vi "rx_adc.vi"(9 "VISA resource name":refnum<visa-resource-name>="COM3", 11 "error in":errorcluster) -> ()   [LabVIEW 2015]
uses:
  <vilib>/Instr/_visa.llb/VISA Configure Serial Port (Instr).vi
  <instrlib>/Rohde&Schwarz RF Signal Generator/Rohde&Schwarz RF Signal Generator.lvlib
panel:
  out "parameters_b":dbl[](array[numeric])
  in  "VISA resource name 2":refnum<visa-resource-name>="GPIB0::28::INSTR" caption="VISA resource name"
  in  "R&S SMA100":refnum<visa-resource-name>="GPIB0::10::INSTR"
  in  "cnt/setp":enum16{"SETP", "COUNT"}(ring)=enum."COUNT"
  out "Freq_Tab":u32[](array[numeric])
  in  "EABLE Insert":bool
  in  "Insert Point":u32
  in  "Value":u32=3 caption="Point Num"
  in  "freq_max(Mhz)":u32=2300
  in  "freq_min(Mhz)":u32=2200
  in  "OK Button":bool
  in  "stop":bool
  in  "Tab Control":enum32{"A通道频谱", "B通道频谱"}(tab)
  out "XY Graph":cluster{dbl[], dbl[]}(graph)
  out "XY Graph 2":cluster{dbl[], dbl[]}(graph)
  out "vol20":string
  out "vol13":string
  out "frequency":string
  out "spectrum_a":dbl[](array[numeric])
  out "fre_a":dbl[](array[numeric])
  out "parameters_a":dbl[](array[numeric])
  out "dBFS_a":dbl
  out "snr_a":dbl
  out "sfdr_a":dbl
  out "sinad_a":dbl
  out "thd_a":dbl
  out "enob_a":dbl
  out "offset_a":dbl
  in  "图片保存路径":path=path "C:/Users/pigandhome/Desktop/Everst_LV2015/Everst_TestReport/Screenshot/RX"
  in  "fifo文件路径":path=path "E:/fifo.txt"
  in  "SPUR340 2":dbl=1.0
  in  "DATA_IQ 2":dbl=1.0
  in  "DATA_LOAD 2":dbl=1.0
  in  "DATA_WRITE 2":dbl=1.0
  in  "NF_TEST 2":dbl
  in  "FFT 2":dbl=1.0
  in  "ANALYZE_INL 2":dbl
  in  "ANALYZE_SPECTRUM 2":dbl=1.0
  in  "NCO 2":dbl=1.0
  in  "CHB":dbl
  out "VISA resource name out":refnum<visa-resource-name>
  in  "FPGA_PHASE":dbl
  in  "LVDS_SELF":dbl
  in  "LOOP_TEST":dbl
  in  "ADC_ONLY":dbl
  in  "STG2":dbl
  in  "STG1":dbl
  in  "CAP_MISMATCH":dbl
  in  "COMP_TRIM":dbl=1.0
  in  "MANUAL_TRIM":dbl=1.0
  in  "PROBE":dbl
  in  "CONFIG_DC":dbl=1.0
  in  "HIZ_INPUT":dbl=1.0
  in  "NCO":dbl=1.0
  in  "CONFIG":bool
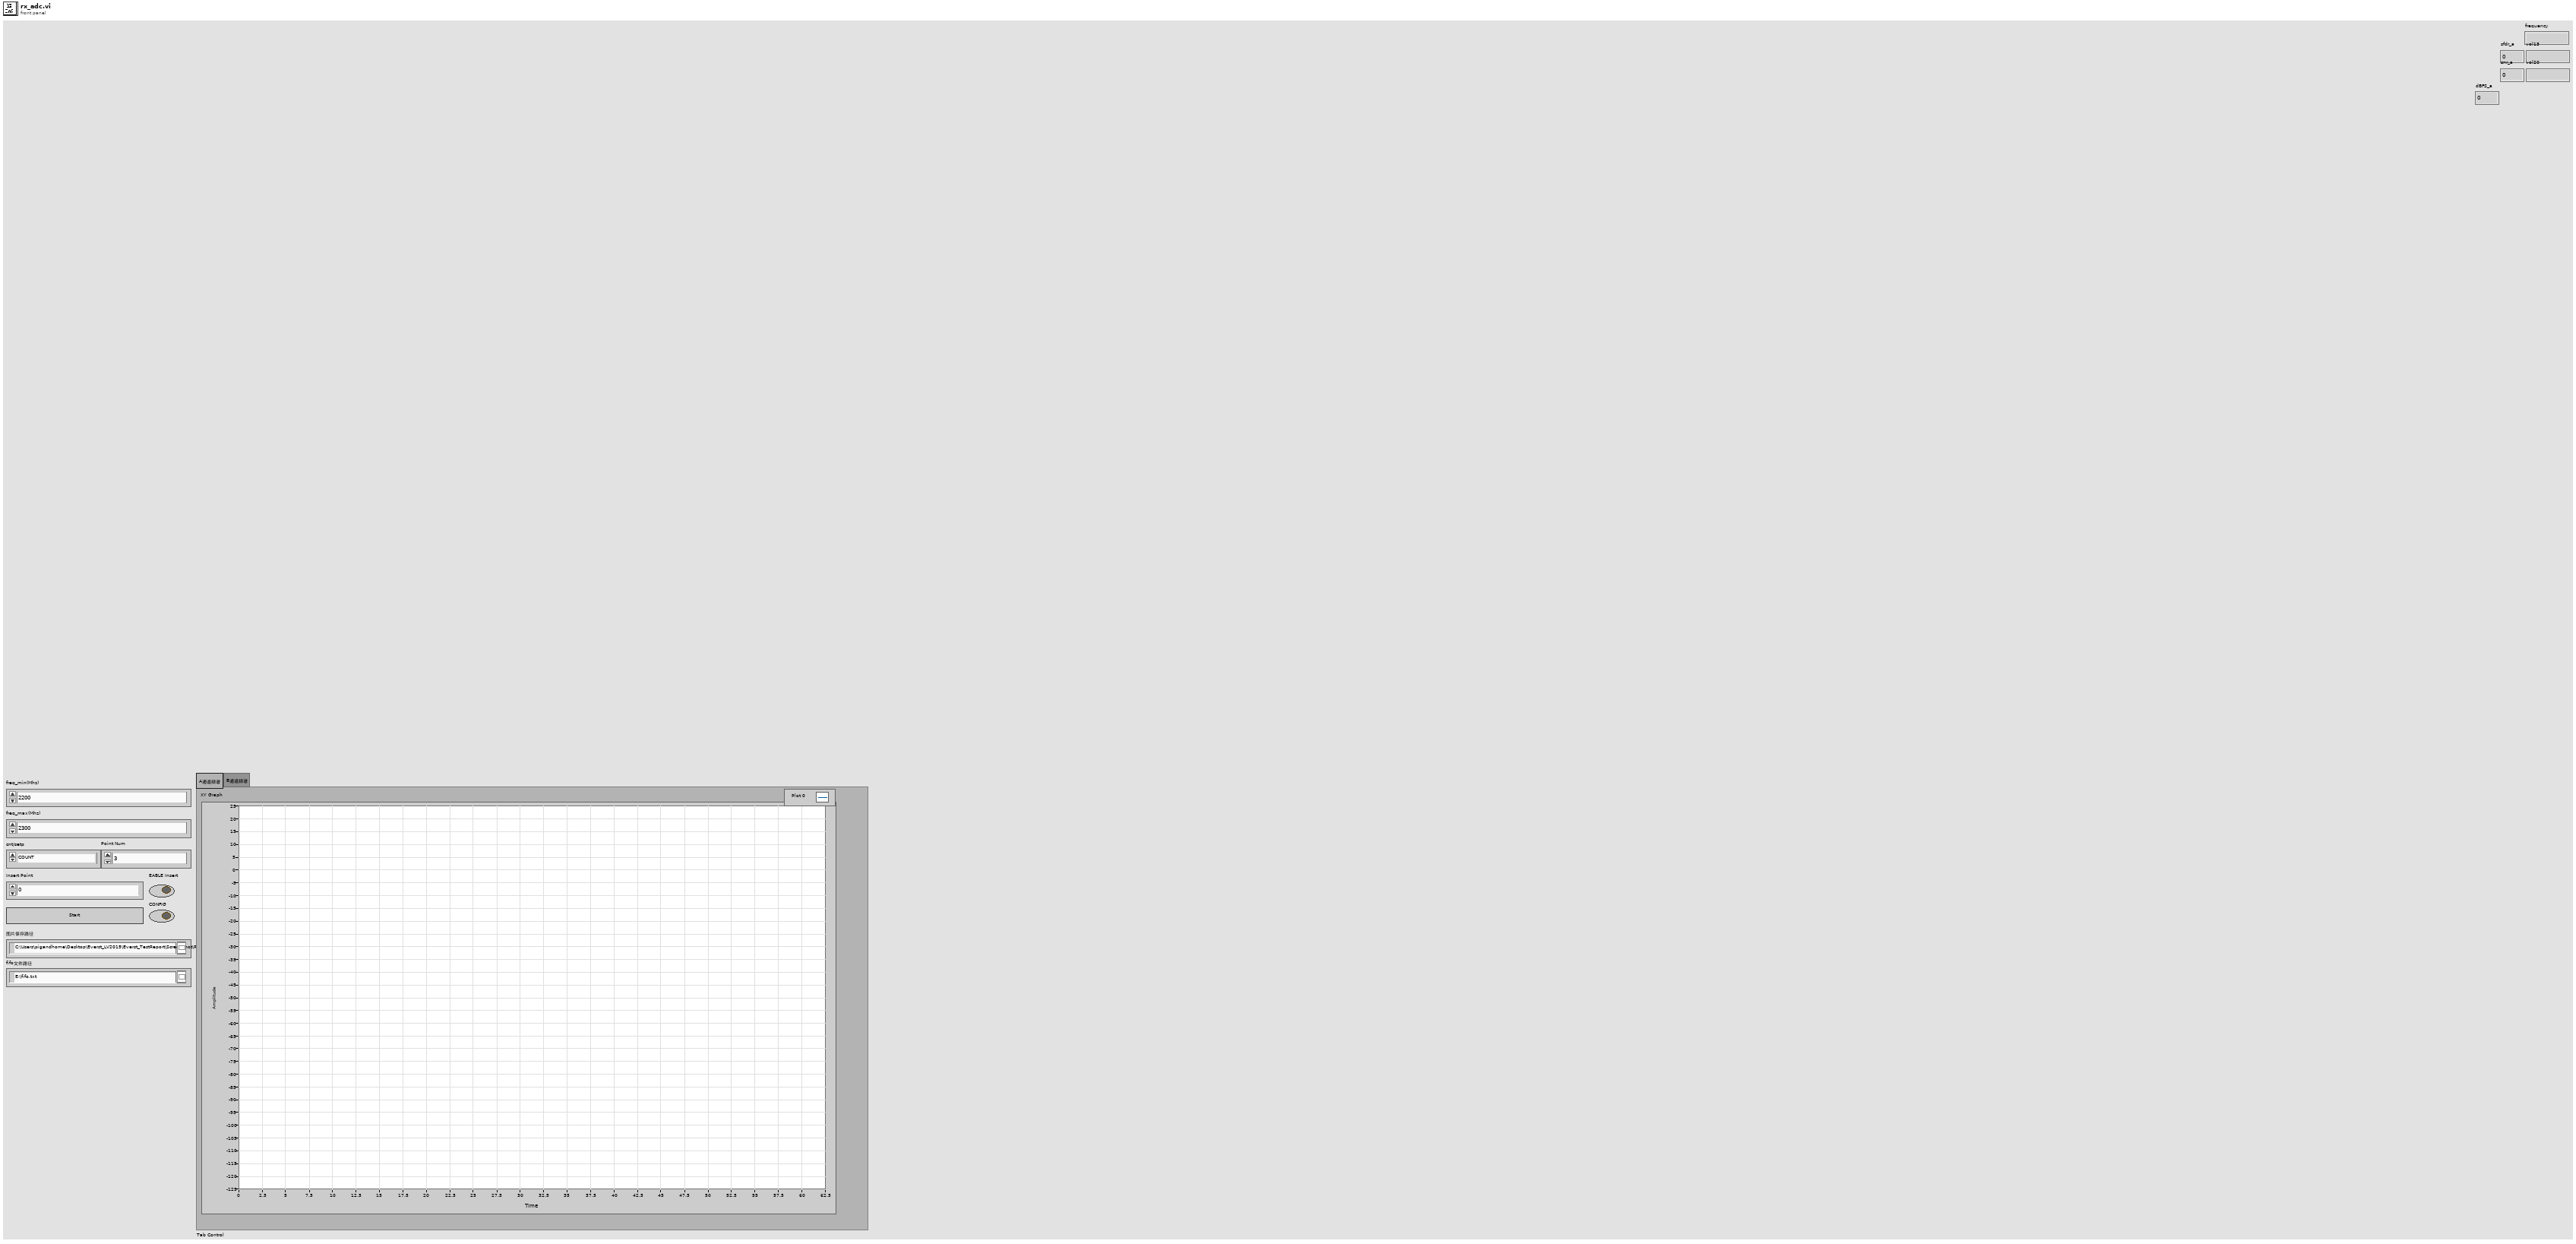
[diagram p1: front panel]
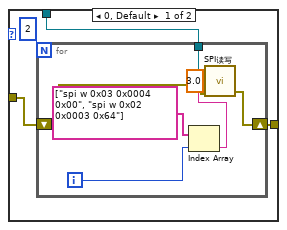
[diagram p3: hidden frame]
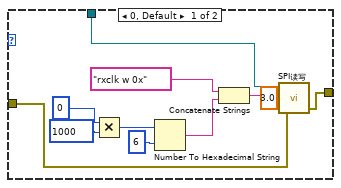
[diagram p4: hidden frame]
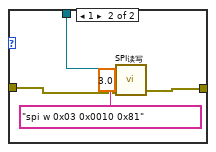
[diagram p5: hidden frame]
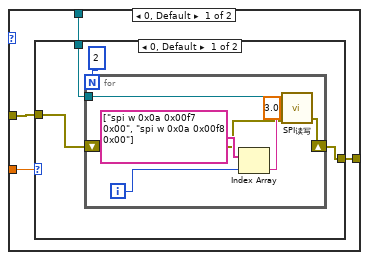
[diagram p6: hidden frame]
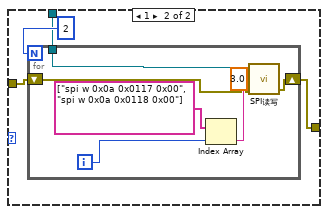
[diagram p7: hidden frame]
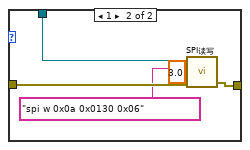
[diagram p10: hidden frame]
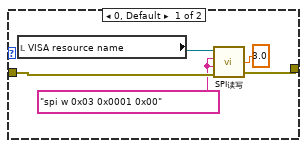
[diagram p12: hidden frame]
diagram:
  w39 = u16 0 items=["无", "XON/XOFF", "RTS/CTS", "XON/XOFF & RTS/CTS", "DTR/DSR", "XON/XOFF & DTR/DSR"] ("flow control (0:none)")
  w40 = u16 10 items=["1.0"=10, "1.5"=15, "2.0"=20] ("stop bits (10: 1 bit)")
  n1 = call-poly "VISA Configure Serial Port"("VISA resource name"="VISA resource name", "baud rate (9600)"=u32 921600, "data bits (8)"=u16 8, "parity (0:none)"=enum16{"None", "Odd", "Even", "Mark", "Space"}."None", "error in (no error)"="error in", "stop bits (10: 1 bit)"=w40, "flow control (0:none)"=w39) -> ("VISA resource name out"=w38:refnum<visa-resource-name>, "error out"=w37:errorcluster)  [unwired: 7 in]
  "VISA resource name out" <- w38
  n2 = VISA Clear(VISA resource name=w38, error in (no error)=w37) -> (VISA resource name out=w34:refnum<visa-resource-name>, error out=w15:errorcluster)
  n3 = call <instrlib>:"RSSMA Initialize.vi"("error in (no error)"=w15, "Resource Name (GPIB::28)"="R&S SMA100") -> ("error out"=w21:errorcluster, "dup VISA session"=w23:refnum<visa-resource-name>)  [unwired: 8 in]
  n4 = call <instrlib>:"RSSMA Configure RF Frequency.vi"("error in (no error)"=w21, "VISA session"=w23) -> ("error out"=w20:errorcluster, "dup VISA session"=w24:refnum<visa-resource-name>)  [unwired: 8 in]
  n5 = call <instrlib>:"RSSMA Configure Fixed RF Level.vi"("VISA session"=w24, "Amplitude (-30.0 dBm)"=-50.0, "error in (no error)"=w20) -> ("dup VISA session"=w18:refnum<visa-resource-name>, "error out"=w19:errorcluster)  [unwired: 11 in]
  n6 = call <instrlib>:"RSSMA Set Output State.vi"("error in (no error)"=w19, "RF Output State (F: Off)"=TRUE, "VISA session"=w18) -> ("error out"=w13:errorcluster, "dup VISA session"=w5:refnum<visa-resource-name>)  [unwired: 7 in]
  n7 = call <instrlib>:"Initialize.vi"("VISA resource name"="VISA resource name 2", "error in (no error)"=w13) -> ("VISA resource name out"=w11:refnum<visa-resource-name>, "error out"=w12:errorcluster)  [unwired: 12 in]
  n8 = call <instrlib>:"Configure RF.vi"("Power Level (-30.0)"=-50.0, "error in"=w12, "Frequency (1.0e9)"=2000000000.0, "VISA resource name"=w11) -> ("error out"=w10:errorcluster, "VISA resource name out"=w9:refnum<visa-resource-name>)  [unwired: 6 in]
  n9 = call <instrlib>:"Configure Output Enabled.vi"("error in"=w10, "Output Enabled (Off)"=TRUE, "VISA resource name"=w9) -> ("error out"=w6:errorcluster, "VISA resource name out"=w4:refnum<visa-resource-name>)  [unwired: 7 in]
  n10 = call "Set_Freq_Table.vi"("EABLE Insert"="EABLE Insert", "Insert Point"="Insert Point", "Value"="Value", "cnt/setp"="cnt/setp", "freq_max(Mhz)"="freq_max(Mhz)", "freq_min(Mhz)"="freq_min(Mhz)") -> ("Freq_Tab"=w2:u32[])
  "Freq_Tab" <- w2
  n11 = Array Size(array=w2) -> (size(s)=w25:i32)
  n12 = while {
    tunnel: w34 -> [w53]
    tunnel: w6 -> [w52]
    tunnel: "fifo文件路径" -> [w50]
    tunnel: "图片保存路径" -> [w49]
    tunnel: w25 -> [w48]
    tunnel: w5 -> [w47]
    tunnel: w4 -> [w46]
    tunnel: w2 -> [w45]
    tunnel: path "C:/Users/pigandhome/Desktop/Everst_LV2015/Everst_TestReport/EVERST_TestReport_#  4_20171014120206.xlsx" ("path") -> [w44]
    stop <- "stop" stop-if-true
    n13 = event shown="[0] \"OK Button\": Value Change" {
      selector: _ -> [_]
      dyn-events: _ -> [_]
      timeout: _ -> [_]
      tunnel: w53 -> [w75]
      tunnel: w52 -> [w74]
      tunnel: w50 -> [w71]
      tunnel: w49 -> [w70]
      tunnel: w48 -> [w69]
      tunnel: w47 -> [w67]
      tunnel: w46 -> [w66]
      tunnel: w45 -> [w60]
      tunnel: w44 -> [w55]
      event "OK Button": Value Change {
        n14 = event-data() -> ()  [unwired: 1 in, 6 out]
        n15 = local read "NCO"() -> (w80:dbl)
        n16 = case shown="1" w80 {
          tunnel: w74 -> [w279 w284]
          tunnel: [w278 w282] -> w76
          frame 0, Default {
            w277 = "spi w 0x03 0x0001 0x00" ("往芯片写数据")
            n17 = local read "VISA resource name"() -> (w280:refnum<visa-resource-name>)
            n18 = call "SPI读写.vi"("DELAY"=3.0, "error in (no error)"=w279, "从芯片读数据"=w277, "往芯片写数据"=w277, "VISA resource name"=w280) -> ("error out"=w278:errorcluster)  [unwired: 1 out]
          }
          frame 1 {
            n19 = local read "VISA resource name"() -> (w285:refnum<visa-resource-name>)
            n20 = call "SPI读写.vi"("DELAY"=3.0, "error in (no error)"=w284, "往芯片写数据"="spi w 0x03 0x0001 0x80", "VISA resource name"=w285) -> ("error out"=w282:errorcluster)  [unwired: 1 in, 1 out]
          }
        }
        n21 = local read "CONFIG"() -> (w77:bool)
        n22 = case shown="True" w77 {
          tunnel: w76 -> [w143 _]
          tunnel: [w143 w166] -> w78
          tunnel: [w142 w144] -> w79
          tunnel: w75 -> [w142 w144]
          frame False {
          }
          frame True {
            w146 = string[] ["spi w 0x08 0x0001 0xe0", "spi w 0x03 0x0005 0x00", "spi w 0x04 0x0000 0x00", "spi w 0x04 0x0001 0x00", "spi w 0x04 0x0002 0x00", "spi w 0x04 0x0000 0x44", "spi w 0x04 0x0001 0x60", "spi w 0x04 0x0002 0x00", "spi w 0x04 0x0005 0x76", "spi w 0x04 0x0006 0x67", "spi w 0x04 0x0007 0x66", "spi w 0x05 0x000e 0x40", "spi w 0x04 0x001c 0x20", "spi w 0x05 0x0003 0xe0", "spi w 0x05 0x0004 0x1f", "spi w 0x05 0x000a 0x20", "spi w 0x05 0x0008 0xe2", "spi w 0x05 0x0008 0xea", "spi w 0x05 0x0015 0x20", "spi w 0x05 0x0016 0x12", "spi w 0x05 0x001c 0x20", "spi w 0x05 0x001a 0xc2", "spi w 0x05 0x001a 0xca", "spi w 0x06 0x000a 0x00", "spi w 0x06 0x0010 0x00", "spi w 0x0a 0x0132 0x5b", "spi w 0x08 0x0012 0x5b", "spi w 0x0a 0x0133 0x71", "spi w 0x08 0x0013 0x71", "spi w 0x06 0x000b 0x3a", "spi w 0x06 0x0003 0x03", "spi w 0x06 0x0009 0xC6", "spi w 0x06 0x0006 0x53", "spi w 0x06 0x0007 0x2E"] ("output array")
            n23 = Array Size(array=w146) -> (size(s)=w148:i32)
            n24 = for {
              N: w148 -> [_]
              tunnel: w146 -> [w173]
              tunnel: w144 -> [w168]
              shift-right: [w167] -> w145
              shift-left: _ -> [w170]
              i -> [w172]
              n25 = Index Array(array=w173, index=w172) -> (element=w171:string)
              n26 = call "SPI读写.vi"("DELAY"=3.0, "error in (no error)"=w170, "从芯片读数据"=w171, "往芯片写数据"=w171, "VISA resource name"=w168) -> ("error out"=w167:errorcluster)  [unwired: 1 out]
            }
            n27 = local read "CONFIG_DC"() -> (w165:dbl)
            n28 = case shown="1" w165 {
              tunnel: w145 -> [w272 w275]
              tunnel: w144 -> [_ w274]
              tunnel: [w272 w273] -> w163
              frame 0, Default {
              }
              frame 1 {
                n29 = call "everest_adc_bias_init.vi"("error in"=w275, "VISA resource name"=w274) -> ("error out"=w273:errorcluster)  [unwired: 9 in]
              }
            }
            n30 = local read "HIZ_INPUT"() -> (w164:dbl)
            n31 = case shown="0, Default" w164 {
              tunnel: w144 -> [w265 w271]
              tunnel: w163 -> [w266 w270]
              tunnel: [w263 w268] -> w161
              frame 0, Default {
                n32 = call "SPI读写.vi"("DELAY"=3.0, "error in (no error)"=w266, "往芯片写数据"="spi w 0x0a 0x0130 0x04", "VISA resource name"=w265) -> ("error out"=w263:errorcluster)  [unwired: 1 in, 1 out]
              }
              frame 1 {
                n33 = call "SPI读写.vi"("DELAY"=3.0, "error in (no error)"=w270, "往芯片写数据"="spi w 0x0a 0x0130 0x06", "VISA resource name"=w271) -> ("error out"=w268:errorcluster)  [unwired: 1 in, 1 out]
              }
            }
            n34 = local read "MANUAL_TRIM"() -> (w162:dbl)
            n35 = case shown="1" w162 {
              tunnel: "CHB" -> [_ w260]
              tunnel: w161 -> [w257 w261]
              tunnel: w144 -> [_ w259]
              tunnel: [w257 w258] -> w159
              frame 0, Default {
              }
              frame 1 {
                n36 = call "everest_adc_manul_trim.vi"("error in (no error)"=w261, "CHB"=w260, "VISA resource name"=w259) -> ("error out"=w258:errorcluster)
              }
            }
            n37 = local read "CAP_MISMATCH"() -> (w160:dbl)
            n38 = local read "STG2"() -> (w157:dbl)
            n39 = local read "STG1"() -> (w158:dbl)
            n40 = case shown="1" w160 {
              tunnel: w159 -> [w250 w256]
              tunnel: w144 -> [_ w255]
              tunnel: "CHB" -> [_ w254]
              tunnel: w158 -> [_ w253]
              tunnel: w157 -> [_ w252]
              tunnel: [w250 w251] -> w155
              frame 0, Default {
              }
              frame 1 {
                n41 = call "everest_adc_cap_mismatch.vi"("STG2"=w252, "STG1"=w253, "error in (no error)"=w256, "CHB"=w254, "VISA resource name"=w255) -> ("error out"=w251:errorcluster)
              }
            }
            n42 = local read "COMP_TRIM"() -> (w156:dbl)
            n43 = case shown="1" w156 {
              tunnel: [w220 w247] -> w153
              tunnel: "CHB" -> [w223 w249]
              tunnel: w144 -> [w222 w248]
              tunnel: w155 -> [w221 w246]
              frame 0, Default {
                n44 = case shown="0, Default" w223 {
                  tunnel: w222 -> [w227 w237]
                  tunnel: w221 -> [w226 w235]
                  tunnel: [w225 w236] -> w220
                  frame 0, Default {
                    n45 = for {
                      N: 2 -> [_]
                      tunnel: w227 -> [w231]
                      shift-right: [w229] -> w225
                      shift-left: w226 -> [w230]
                      i -> [w234]
                      n46 = Index Array(array=string[] ["spi w 0x0a 0x00f7 0x00", "spi w 0x0a 0x00f8 0x00"], index=w234) -> (element=w232:string)
                      n47 = call "SPI读写.vi"("DELAY"=3.0, "error in (no error)"=w230, "往芯片写数据"=w232, "VISA resource name"=w231) -> ("error out"=w229:errorcluster)  [unwired: 1 in, 1 out]
                    }
                  }
                  frame 1 {
                    n48 = for {
                      N: 2 -> [_]
                      shift-right: [w241] -> w236
                      shift-left: w235 -> [w242]
                      tunnel: w237 -> [w240]
                      i -> [w245]
                      n49 = Index Array(array=string[] ["spi w 0x0a 0x0117 0x00", "spi w 0x0a 0x0118 0x00"], index=w245) -> (element=w243:string)
                      n50 = call "SPI读写.vi"("DELAY"=3.0, "error in (no error)"=w242, "往芯片写数据"=w243, "VISA resource name"=w240) -> ("error out"=w241:errorcluster)  [unwired: 1 in, 1 out]
                    }
                  }
                }
              }
              frame 1 {
                n51 = call "everest_adc_comp_trim_init.vi"("CHB"=w249, "error in (no error)"=w246, "VISA resource name"=w248) -> ("error out"=w247:errorcluster)
              }
            }
            n52 = local read "LVDS_SELF"() -> (w154:dbl)
            n53 = case shown="0, Default" w154 {
              tunnel: w153 -> [w212 w218]
              tunnel: w144 -> [w213 w217]
              tunnel: [w211 w216] -> w151
              frame 0, Default {
                n54 = call "SPI读写.vi"("DELAY"=3.0, "error in (no error)"=w212, "往芯片写数据"="spi w 0x03 0x0010 0x80", "VISA resource name"=w213) -> ("error out"=w211:errorcluster)  [unwired: 1 in, 1 out]
              }
              frame 1 {
                n55 = call "SPI读写.vi"("DELAY"=3.0, "error in (no error)"=w218, "往芯片写数据"="spi w 0x03 0x0010 0x81", "VISA resource name"=w217) -> ("error out"=w216:errorcluster)  [unwired: 1 in, 1 out]
              }
            }
            n56 = local read "FPGA_PHASE"() -> (w152:dbl)
            n57 = case shown="1" w152 {
              tunnel: w151 -> [w191 w202]
              tunnel: w144 -> [w190 w201]
              tunnel: [w189 w200] -> w149
              frame 0, Default {
                n58 = Multiply(x=0, y=1000) -> (x*y=w196:i32)
                n59 = Number To Hexadecimal String(1:i16 6 ("宽度(-)"), 2:w196) -> (0:w193:string)
                n60 = Concatenate Strings("rxclk w 0x", w193) -> (w192:string)
                n61 = call "SPI读写.vi"("DELAY"=3.0, "error in (no error)"=w191, "往芯片写数据"=w192, "VISA resource name"=w190) -> ("error out"=w189:errorcluster)  [unwired: 1 in, 1 out]
              }
              frame 1 {
                n62 = Multiply(x=90, y=1000) -> (x*y=w207:i32)
                n63 = Number To Hexadecimal String(1:i16 6 ("宽度(-)"), 2:w207) -> (0:w204:string)
                n64 = Concatenate Strings("rxclk w 0x", w204) -> (w203:string)
                n65 = call "SPI读写.vi"("DELAY"=3.0, "error in (no error)"=w202, "往芯片写数据"=w203, "VISA resource name"=w201) -> ("error out"=w200:errorcluster)  [unwired: 1 in, 1 out]
              }
            }
            n66 = local read "LOOP_TEST"() -> (w150:dbl)
            n67 = case shown="1" w150 {
              tunnel: w149 -> [w176 w186]
              tunnel: w144 -> [w175 w187]
              tunnel: [w174 w185] -> w166
              frame 0, Default {
                n68 = for {
                  N: 2 -> [_]
                  tunnel: w175 -> [w180]
                  shift-right: [w179] -> w174
                  shift-left: w176 -> [w181]
                  i -> [w184]
                  n69 = Index Array(array=string[] ["spi w 0x03 0x0004 0x00", "spi w 0x02 0x0003 0x64"], index=w184) -> (element=w182:string)
                  n70 = call "SPI读写.vi"("DELAY"=3.0, "error in (no error)"=w181, "往芯片写数据"=w182, "VISA resource name"=w180) -> ("error out"=w179:errorcluster)  [unwired: 1 in, 1 out]
                }
              }
              frame 1 {
                n71 = call "everest_loop_test.vi"("error in (no error)"=w186, "VISA resource name"=w187) -> ("error out"=w185:errorcluster)
              }
            }
          }
        }
        n72 = VISA Close(VISA resource name=w79, error in (no error)=w78) -> (error out=w68:errorcluster)
        n73 = Path To String(path=w71) -> (string=w72:string)
        n74 = Path To String(path=w70) -> (string=w73:string)
        n75 = for {
          N: w69 -> [_]
          tunnel: w73 -> [w112]
          tunnel: w72 -> [w111]
          shift-right: [w110] -> _
          shift-left: w68 -> [w109]
          tunnel: w67 -> [w107]
          tunnel: w66 -> [w106]
          tunnel: [w87] -> w58 mode=indexing
          tunnel: [w83] -> w57 mode=indexing
          i -> [w104]
          n76 = local read "Freq_Tab"() -> (w105:u32[])
          n77 = local read "frequency"() -> (w126:string)
          n78 = local read "vol13"() -> (w127:string)
          n79 = local read "vol20"() -> (w128:string)
          n80 = Index Array(array=w105, index=w104) -> (element=w92:u32)
          n81 = Less?(x=w92, y=u32 2270) -> (x < y?=w88:bool)
          n82 = Boolean To (0,1)(Boolean=w88) -> (0, 1=w89:i16)
          n83 = Multiply(x=u32 1000000, y=w92) -> (x*y=w101:u32)
          n84 = call <instrlib>:"RSSMA Configure RF Frequency.vi"("error in (no error)"=w109, "Frequency (1.0e9 Hz)"=w101, "VISA session"=w107) -> ("error out"=w108:errorcluster)  [unwired: 7 in, 1 out]
          n85 = script code="if ANALYZE_SPECTRUM\n    fifo_len = 31;   %%% unit is k, 16/32/63\nelse\n    fifo_len = 16;   %%% unit is k\nend % ANALYZE_SPECTRUM\n%--------------------------------------------------------------------------\nfile = path;\n%--------------------------------------------------------------------------\n\nif CHB\n    file_captrim = 'chip2_chb_cap.mat';\nelse\n    file_captrim = 'chip2_cha_cap.mat';\nend % CHB\n%--------------------------------------------------------------------------\n\n%Initial s port\ns         = serial('COM3');     % need to change if com number changes\ns.InputBufferSize = 128e3;\nset(s,'BaudRate',921600);\nfopen(s);\n\n\nif ANALYZE_SPECTRUM\n\n    if DATA_WRITE\n%        fifo_data = fifo_read(s, fifo_len);\ncommand = sprintf('fifo rst\\n');\nfwrite(s, command);\nfprintf('%s',command);\npause(0.1);\ncommand = sprintf('fifo rst\\n');\nfwrite(s, command);\nfprintf('%s',command);\npause(0.1);\ncommand = sprintf('fifo status\\n');\nfwrite(s,command);\nfprintf('%s',command);\npause(0.03);\ncommand = sprintf('fifo wr\\n');\nfwrite(s,command);\npause(1);\ncommand = sprintf('fifo status\\n');\nfwrite(s,command);\npause(0.03);\ncommand = sprintf('fifo read 0x%s\\n',dec2hex(fifo_len,2));\nfwrite(s,command);\npause(0.03);\n\npause(0.03);\nnum1 = s.BytesAvailable;\n\ndata_buffer = int8(zeros(1,fifo_len*1e3*30+500));\nfprintf(1,'Read fifo(%dK).',fifo_len);\n\nii = 1;\nwhile num1 ~= 0\n    pause(0.1);    \n    read_data = fread(s, num1);\n    data_buffer(ii:ii+num1-1) = read_data';\n    ii = ii + num1;\n    num1 = s.BytesAvailable;\n    fprintf(1,'.');\n%     fprintf(1,'%d\\n',ii);\nend\n\nfprintf(1,'\\n');\nfifo_data = data_buffer;\n\n       fprintf(1,'---------------------Read fifo ok!------------------------------\\n');\n       fid = fopen(file,'w');\n       fprintf(fid,'%1c',fifo_data);\n       fclose(fid);\n    end\n\n    fclose(s);\n%--------------------------------------------------------------------------\n    if DATA_LOAD\n    % read from data file\n    fid      = fopen(file,'r');\n    temp     = fscanf(fid, '%s'); \n    len_temp = length(temp);\n\n    for ii = 1:1:3000\n       if strcmp(temp(ii:ii+9),'fiforead0x')\n           break;\n       end\n    end\n\n    temp1              = temp(ii+12:fifo_len*16*1024+ii+11);\n    num_of_samples     = length(temp1)/16;\n\n    samples_rising_a   = zeros(1,num_of_samples);\n    samples_falling_a  = zeros(1,num_of_samples);\n\n    samples_rising_b   = zeros(1,num_of_samples);\n    samples_falling_b  = zeros(1,num_of_samples);\n\n    for ii = 1:1:num_of_samples\n        temp_rising_a  = temp1(((ii-1)*16+1):((ii-1)*16+4));\n        temp_falling_a = temp1((ii-1)*16+5:(ii-1)*16+8);\n        temp_rising_b  = temp1((ii-1)*16+9:(ii-1)*16+12);\n        temp_falling_b = temp1((ii-1)*16+13:(ii-1)*16+16);\n\n        samples_rising_a(ii)   = hex2dec(temp_rising_a);\n        samples_falling_a(ii)  = hex2dec(temp_falling_a);\n        samples_rising_b(ii)   = hex2dec(temp_rising_b);\n        samples_falling_b(ii)  = hex2dec(temp_falling_b);\n\n        if samples_rising_a(ii) > 2^13-1\n            samples_rising_a(ii) = samples_rising_a(ii) - 2^14;\n        end\n\n        if samples_rising_b(ii) > 2^13-1\n            samples_rising_b(ii) = samples_rising_b(ii) - 2^14;\n        end\n\n        if samples_falling_a(ii) > 2^13-1\n            samples_falling_a(ii) = samples_falling_a(ii) - 2^14;\n        end\n\n        if samples_falling_b(ii) > 2^13-1\n            samples_falling_b(ii) = samples_falling_b(ii) - 2^14;\n        end\n    end\n\n    mean_rising_a   = round(mean(samples_rising_a));\n    mean_falling_a  = round(mean(samples_falling_a));\n    mean_rising_b   = round(mean(samples_rising_b));\n    mean_falling_b  = round(mean(samples_falling_b));\n    end \n\n    fclose all;\n%--------------------------------------------------------------------------\n\n% % plot data\n% figure('name','sampled waveform');\n% \n% subplot(2,2,1); \n% plot(samples_rising_a); \n% title('ADC VI output'); \n% grid on;\n% hold on;\n% \n% subplot(2,2,2);\n% plot(samples_falling_a);\n% title('ADC VQ output');\n% grid on;\n% hold on;\n% \n% subplot(2,2,3); \n% plot(samples_rising_b);\n% title('ADC HI output');\n% grid on;\n% hold on;\n% \n% subplot(2,2,4);\n% plot(samples_falling_b);\n% title('ADC HQ output');\n% grid on;\n% hold on;\n%--------------------------------------------------------------------------\n\n% do fft analysis\nif FFT\n\n    if CHB    % CHB\n        dataI = samples_rising_b';\n        dataQ = samples_falling_b';\n        \n        if NCO\n            if DATA_IQ\n                data  = dataI - j*dataQ;\n            else\n                data  = dataQ - j*dataI;\n            end\n        else\n            data  = dataQ;\n        end\n        \n    else      % CHA\n        dataI = samples_rising_a';\n        dataQ = samples_falling_a';\n   \n        if NCO\n            if DATA_IQ\n                data  = dataI - j*dataQ;\n            else\n                data  = dataQ - j*dataI;\n            end\n        else\n            data  = dataQ;\n        end\n    end\n\n    if NF_TEST\n        len  = length(data); \n        fs   = 125e6; \n        fsig = 5e6;\n        t    = 1/fs:1/fs:len/fs; \n        %sig  = 8191*cos(2*pi*t*fsig);\n        sig  = 8191*cos(2*pi*t*fsig) + j * 8191*cos(2*pi*t*fsig);\n        data = data + sig';\n    end\n    \n    if SPUR340\n        len  = length(data); \n        fs   = 125e6; \n        fsig = 20e6;\n        t    = 1/fs:1/fs:len/fs;\n        amp  = 8191 * 10^(-59.2198/20);\n        td   = 0 ;\n        phase = 0.0717;\n        %sig  = 8191*cos(2*pi*t*fsig);\n        sig  = amp*cos(2*pi*(t+td)*fsig+phase) - j * amp*sin(2*pi*(t+td)*fsig+phase);\n        win  = hanning(len);\n        data_fft  =  fft(data.*win);\n        sig_fft   =  fft(sig'.*win);\n        abs(data_fft(5244))\n        abs(sig_fft(5244))\n        angle(data_fft(5244))\n        angle(sig_fft(5244))\n        %data = data - sig';   \n    end\n    \n    save fftdata.dat data -ASCII\n\n%     Dynamics_14b_no_print;\n%Filename:   Dynamics_12b.m\n%Function:   Spectrum analaysis of 12b ADC\n%Author:     Maxgress\n%Date:       Dec. 2012\n%--------------------------------------------------------------------------\n\n%set constants\n%--------------------------------------------------------------------------\n\n%fsample  = 61.44e6*4;           % clock frequency\nfsample  = 500e6/4;           % clock frequency\nfsr      = 1;\n%numpts   = 131072*2;          % 128k data\nnumpts   = 4096;            % 128k data\nnumbits  = 14;              % 12bit \nsearch   = 1;                      \nnumharm  = 3;              % Number of harmonics \n\n\n%load data\n%--------------------------------------------------------------------------\n\n%load C:\\MG6802\\fftdata.dat;\n%load fftdata.dat\n\n%data     = fftdata;\n[a b]    = size(data);\nnumpts   = a;\nwindow   = 1;\ntwotone  = 0;\ndither   = 0;\n\n%dBFS     = 20*log10((max(real(data))-min(real(data)))/2^numbits);\ndBFS     = 10*log10(((max(real(data))-min(real(data)))/2^numbits)^2 + ((max(imag(data))-min(imag(data)))/2^numbits)^2);\n\ntmp1     = size(data);\ntmp1     = tmp1(1);\n\n%process data\n%--------------------------------------------------------------------------\n\nq        =  data;\nfbin     = (fsample/numpts);\t%this is the the FFT bin spacing\nVopp     =  max(q)-min(q);\t%this is the Peak-to-Peak ADC output\nVodbfs   =  20*log10(Vopp/2);\t%this is the ADC output in dBFS\nshift    =  (2^(numbits-1))-0.5;\nu        =  (q-shift)/shift;\n\nz        =   fft(u)/numpts;\n\n%%%%%%%%% Here are some magic windowing factors \n\nif window==1;\n   a0=0.3635819;\n   a1=0.4891775;\n   a2=0.1365995;\n   a3=0.0106411;\n   vec=0.5*[-a3 a2 -a1 2*a0 -a1 a2 -a3]*(numpts/2^numbits);\n   winh=conv(vec,z);\n   for i=1:numpts;\n\t\tz(i)=winh(i+3);\n   end;\n\t\t\nend;\nGwin=-20*log10(a0);\t     %this is the window's gain\n\n%%%%%%%%%  these simple transforms are how we use the fft result:\n\nvolts=abs(z(1:(numpts/2+1)));\n%volts(numpts/4:numpts/2+1)=0.00001;\n\npower=volts.^2;\ndbvolts=20*log10(2*volts+eps); % Why the factor of 2 applied to volts.\n%dbvolts(numpts/4:numpts/2+1)=-92;\nif window==1;\n\tdbvolts=dbvolts+Gwin;\t%this resets to normalized gain\nend;\ndbint=floor(dbvolts);\n\n%  if the oscillator frequencies are all over the place,\n%  we can go and find the input by looking for the max \n%  bin.  This is selected by the \"search\" flag.\n\nif search==1\n\ttempvolts=volts;\n\ttempvolts(1:4)=zeros(1,4);\n\t[a1,fund]=max(tempvolts);\n   finput=(fund-1)*fsample/numpts;\n   tempvolts(fund)=0;\n   if(twotone==1)\n      [a2,fundq]=max(tempvolts);\n      finputq=(fundq-1)*fsample/numpts;\n   end;   \nend;\n\n%%%%%%%%%%%%%  Now we analyze the results of the fft;\n%%%%%%%%%%%%%  If we know finput, we can find the harmonics:\nif(twotone==1)\nhq=0:(numharm-1);\nfhq=finputq*hq;\nrbinsq=round(fhq/(fsample/numpts));\nmultq=(floor(rbinsq/(numpts/2)));\npolq=(-1).^multq;\nactbinq=1+(numpts/2)*(1-polq)/2+polq.*(rbinsq-multq*numpts/2);\nfor i=1:numharm;\n      hdarrayq(i)=dbvolts(actbinq(i));\nend;\nend;\n\nh=0:(numharm-1);\nfh=finput*h;\nrbins=round(fh/(fsample/numpts));\nmult=(floor(rbins/(numpts/2)));\npol=(-1).^mult;\nactbin=1+(numpts/2)*(1-pol)/2+pol.*(rbins-mult*numpts/2);\ndbvoltsa=dbvolts;\n\nfor i=1:numharm;\n  \n      hdarray(i)=dbvolts(actbin(i));\n\nend;\n\n%%%%%%% After calculating harmonic bin locations, we can calculate the\n%%%%%%% noise floor for the SNR & SINAD. First exclude the power in the  \n%%%%%%% dither (this is the \"dither\" variable) band and the 50 individual\n%%%%%%% harmonic bins and the DC bin. An iterative approach is used.\n%%% actbin(1) is DC bin.  \n%%% actbin(2) is the fundamental.\n\nif dither>0\n\tpbins=power;\n\tstartBin=dither/fbin;\n\tavgpwr1=sum(pbins(startBin+1):pbins(startBin+5));\n\tfor i=1:startBin;\n\t\tpbins(i)=avgpwr1;\n\tend;\nelse\n\tpbins=power;\nend;\nsfdrarray=pbins;\nzeroset=0;\npowleng=1+length(power);\nvart=8;\nif window==0\n   \tfor i=1:numharm;\n         pbins(actbin(i))=0;\n         if(twotone==1)\n            pbins(actbinq(i))=0;\n         end;\n      end;\n\t\t\tavgpwr2=mean(pbins)*((numpts/2)+1)/((numpts/2)-(numharm)+1);\n\t\n   %%%%% Commenting out code which fills harmonic bins with average\n   %%%%% power with window == 0.\n%\tfor i=1:numharm;\n%\t\tpbins(actbin(i))=avgpwr2;\n%\tend;\n\n%%% this next bunch of loops deal with the window's sidelobes\nelse\n\tfor i=1:numharm;\n\t\tif (actbin(i)-4) >  0;\n\t\t\tpbins(actbin(i)-4)=0;\n\t\t\tzeroset=zeroset+1;\n\t\t\tend;\n\t\tif (actbin(i)-3) >  0;\n\t\t\tpbins(actbin(i)-3)=0;\n\t\t\tzeroset=zeroset+1;\n\t\t\tend;\n\t\tif (actbin(i)-2) >  0;\t\n\t\t\tpbins(actbin(i)-2)=0;\n\t\t\tzeroset=zeroset+1;\n\t\t\tend;\n\t\tif (actbin(i)-1) >  0;\t\n\t\t\tpbins(actbin(i)-1)=0;\n\t\t\tzeroset=zeroset+1;\n\t\t\tend;\n\t\tpbins(actbin(i))=0;\n\t\tzeroset=zeroset+1;\n\t\tif (actbin(i)+1) < powleng\n\t\t\tpbins(actbin(i)+1)=0;\n\t\t\tzeroset=zeroset+1;\n\t\t\tend;\n\t\tif (actbin(i)+2) < powleng\n\t\t\tpbins(actbin(i)+2)=0;\n\t\t\tzeroset=zeroset+1;\n\t\t\tend;\n\t\tif (actbin(i)+3) < powleng\n\t\t\tpbins(actbin(i)+3)=0;\n\t\t\tzeroset=zeroset+1;\n\t\t\tend;\n\t\tif (actbin(i)+4) < powleng\n\t\t\tpbins(actbin(i)+4)=0;\n\t\t\tzeroset=zeroset+1;\n\t\t\tend;\n\tend;\n\tavgpwr2=mean(pbins)*(numpts+1)/((numpts)-3-zeroset);\nend;\n\nif dither>0\n\tfor i=1:startBin;\n\t\tpbins(i)=avgpwr2;\n\tend;\nend;\n\nif(window==1)\n\tfor i=1:numharm;\n\t\tif (actbin(i)-4) >  0;\n\t\t\tpbins(actbin(i)-4)=avgpwr2;\n\t\tend;\n\t\tif (actbin(i)-3) >  0;\n\t\t\tpbins(actbin(i)-3)=avgpwr2;\n\t\tend;\n\t\tif (actbin(i)-2) >  0;\t\n\t\t\tpbins(actbin(i)-2)=avgpwr2;\n\t\tend;\n\t\tif (actbin(i)-1) >  0;\t\n\t\t\tpbins(actbin(i)-1)=avgpwr2;\n\t\tend;\n\t\tpbins(actbin(i))=avgpwr2;\n\t\tif (actbin(i)+1) < powleng\n\t\t\tpbins(actbin(i)+1)=avgpwr2;\n\t\tend;\n\t\tif (actbin(i)+2) < powleng\n\t\t\tpbins(actbin(i)+2)=avgpwr2;\n\t\tend;\n\t\tif (actbin(i)+3) < powleng\n\t\t\tpbins(actbin(i)+3)=avgpwr2;\n\t\tend;\n\t\tif (actbin(i)+4) < powleng\n\t\t\tpbins(actbin(i)+4)=avgpwr2;\n\t\tend;\n\tend;\n    %if (actbin(2)-4 < 1) low_lim = 1; else low_lim = actbin(2) - 4; end\n    %if (actbin(2)+4 > length(power)) high_lim = length(power); else high_lim = actbin(2) + 4; end\n    \n    if (actbin(2)- 128 < 1) low_lim = 1; else low_lim = actbin(2) - 128; end\n    if (actbin(2)+ 128 > length(power)) high_lim = length(power); else high_lim = actbin(2) + 128; end\n    \n\tfundpower=sum(power(low_lim:high_lim));\n\tsnr=10*log10(fundpower/sum(pbins));\n\thdarray';\nend;\n\n\n% This one calculates the ADC's thermal noise floor w.r.t. FSR\n%\t\"Gwin\" is the reciprocal of the window's gain\nif window==1\n\tGwin=-1*(20*log10(a0));\nelse\n\tGwin=0;\nend;\nGfft=10*log10(numpts);\nnoisefloor=Gfft + 20*log10(avgpwr2^.5) + Gwin;\n\nif(window==0)\n   if(twotone==1)\n      fundpower=power(actbin(2))+power(actbinq(2));\n   else\n      fundpower=power(actbin(2));\n   end;\n   if(ericsson==1)\n      snr=10*log10(fundpower/sum(pbins(1:1024)))\n   else\n      snr=10*log10(fundpower/sum(pbins))\n   end;\n   \n\thdarray';\nend;\n\nfundampl=hdarray(2);\n\n\n%  Now we use the sfdrarray generated above, remove the fundamental and\n%  bins, and look for\n%  the next largest bin.  We calculate SFDR, then output a number showing\n%  the dominant harmonic\n%  0 will represent a non-harmonic spur...\n\nsfdrarray(1)=0;\nsfdrarray(actbin(2))=0;\nif(twotone==1)\n   sfdrarray(actbinq(2))=0;\nend;\nif window==1;\n\tsfdrarray(1:4)=zeros(1,4);\n\tsfdrarray(low_lim:high_lim)=zeros(1,high_lim-low_lim+1);\nend;\nsfdr_ray=sfdrarray;\n \n[a,sfdrbin]=max(sfdr_ray);\nsfdrbin;\nsfdr=10*log10((power(actbin(2)))/a);\ndomharm=0;\nfor i=3:numharm;\n\tif actbin(i)==sfdrbin;\n\t\tdomharm=i-1;\n\tend;\nend;\ndomharm;\nspurfreq=(sfdrbin-1)*fsample/numpts;\n\n%%%%   SINAD calculation\n%%%%  I think that it is valid to eliminate the dc bin for calculating SINAD.\n%%%%  I need to check\n%%%%  to see if everyone else agrees with this.\n\nif window==0\n\t% sfdrarray(1)=avgpwr2; %Add average noise power to DC bin.\n   if(ericsson==1)\n      allnoise=sum(sfdrarray(1:1024));\n   else\n      allnoise=sum(sfdrarray);\n   end;\n   if(twotone==1)\n      sinad=10*log10((power(actbin(2))+power(actbinq(2)))/allnoise);\n   else\n      sinad=10*log10(power(actbin(2))/allnoise);\n   end;\n   \nelse\n\tsfdrarray(1:4)=avgpwr2*ones(1,4);\n\tallnoise=sum(sfdrarray);\n\tsinad=10*log10(fundpower/allnoise);\nend;\n\nwinharm=[];\n\nif(window==1)\n   winfund=power(low_lim:high_lim);\n   for i=3:numharm;\n      winharm=[winharm power(low_lim:high_lim)'];\n   end;\n   thd=10*log10(sum(winfund)/sum(sum(winharm)));\nelse\n   \n%   Now we want to calculate THD (in dBc).  This is just:\n%Need total Harmonic calculation for window == 1.\n\n\ttotharm=0;\n\tfor i=3:numharm;\n      if(ericsson==1)\n      \tif(actbin(i)>1024)\n         \ttotharm=totharm;\n      \telse\n         \ttotharm=totharm+power(actbin(i));\n      \tend;\n   \telse\n      \ttotharm=totharm+power(actbin(i));\n   \tend;\n\tend;\n\tthd=10*log10(power(actbin(2))/totharm)\n\nend;\n\n%%%%%%%%%%  To check the calculations, I compared the sum of thd and snr to the\n%%%%%%%%%%  sinad=\n%%%%%%%%%%   calculated.  They work out quite closely with various input SNR's.\n\nsinad2=10*log10(1/(10^(thd/10))+1/(10^(snr/10)));\nsinad+sinad2;\n\n%%%%%%%%  ENOB calculation: \n\nenob=(sinad-1.760912)/6.0206;\nHD2=dbvolts(actbin(2))-dbvolts(actbin(3));\n% HD3=dbvolts(actbin(2))-dbvolts(actbin(4));\n\n%  One final calculation: dc offset in mv\n%  note that fsr is the full scale range (peak to peak) in volt\noffset=mean(data);\nxax=fbin*(1:1:numpts/2+1);\nspectrum=dbvolts(10:length(dbvolts));\nspectrum=dbvolts-max(spectrum);\n%offset, fundampl, snr, sfdr, thd, sinad, noisefloor\n\n\n\n    if CHB\n        fprintf(1,'CHB analys \\n dBFs=%4.2fdB  SNR=%4.2fdB  SFDR=%4.2fdB  SINAD=%4.2fdB \\n THD =  %4.2fdB  ENOB=%4.2fbits  OFFSET=%4.2fLSBS\\n',dBFS,snr,sfdr,sinad,thd,enob,offset);\n    else\n        fprintf(1,'CHA analys \\n dBFs=%4.2fdB  SNR=%4.2fdB  SFDR=%4.2fdB  SINAD=%4.2fdB \\n THD =  %4.2fdB  ENOB=%4.2fbits  OFFSET=%4.2fLSBS\\n',dBFS,snr,sfdr,sinad,thd,enob,offset);\n    end\n\nfigure('name','frequency_spectrum');\n\n    freq = linspace(0,numpts/2,numpts/2+1)/numpts * fsample/1e6;\n\nplot(freq,spectrum);\n\nfre_spectrum=spectrum';\n\n    if CHB\n        title('ADC CHB output spectrum(H)'); \n    else\n        title('ADC CHA output spectrum(V)');\n    end\n\nxlabel('Freq(MHz)'); \nnote = sprintf('SNR = %5.2fdB\\nSFDR = %5.2fdB\\ndBFS = %5.2fdB\\n',snr,sfdr,dBFS);\ntext(max(freq)/2,max(spectrum)-30,note);\ngrid on;\n\ntime=datestr(now,'yyyymmddTHHMMSS');\nsaveas(gcf,[path_jpg,'A_',frequency,vol13,vol20,'_',time],'jpg');\n\nfprintf(1,'---------------------FFT analysis done!-------------------------\\n');\n\nend  % if FFT\nelse\nfclose(s);\nend  % if ANALYZE_SPECTRUM\n%--------------------------------------------------------------------------\n\nif ANALYZE_INL\n    DNLINL_14b;\n    figure;\n    plot(INL);\n    fprintf(1,'---------------------INL analysis done!-------------------------\\n');\nend\n%--------------------------------------------------------------------------\n%--------------------------------------------------------------------------"("??"=w82, "ANALYZE_SPECTRUM"=1.0 ("Real"), "DATA_WRITE"=1.0 ("Real"), "DATA_LOAD"=1.0 ("Real"), "CHB"=0.0 ("Real"), "FFT"=0.0 ("Real"), "NCO"=0.0 ("Real"), "DATA_IQ"=w89, "NF_TEST"=0.0 ("Real"), "SPUR340"=1.0 ("Real"), "ANALYZE_INL"=0.0 ("Real"), "path"=w111, "path_jpg"=w112, "frequency"=w126, "vol13"=w127, "vol20"=w128) -> ("??"=w114:errorcluster, "freq"=w131:dbl[], "fre_spectrum"=w130:dbl[], "dBFS"=w136:dbl, "snr"=w135:dbl, "sfdr"=w134:dbl, "sinad"=→"sinad_a":dbl, "thd"=→"thd_a":dbl, "enob"=→"enob_a":dbl, "offset"=→"offset_a":dbl)
          "sfdr_a" <- w134
          "snr_a" <- w135
          "dBFS_a" <- w136
          "fre_a" <- w131
          "spectrum_a" <- w130
          n86 = call <instrlib>:"Configure RF.vi"("Power Level (-30.0)"=-50.0, "error in"=w108, "Frequency (1.0e9)"=w101, "VISA resource name"=w106) -> ("error out"=w81:errorcluster)  [unwired: 6 in, 1 out]
          n87 = flat-sequence {
            tunnel: [w140] -> w82
            tunnel: w81 -> [w140]
            frame #0 {
              n88 = Wait (ms)(milliseconds to wait=u32 1000) -> ()  [unwired: 1 out]
            }
          }
          n89 = Bundle(w131, w130) -> (→"XY Graph":cluster{dbl[], dbl[]})  [unwired: 1 in]
          n90 = Build Array(w136, w135, w134) -> (w87:dbl[])
          "parameters_a" <- w87
          n91 = Boolean To (0,1)(Boolean=w88) -> (0, 1=w90:i16)
          n92 = script code="if ANALYZE_SPECTRUM\n    fifo_len = 31;   %%% unit is k, 16/32/63\nelse\n    fifo_len = 16;   %%% unit is k\nend % ANALYZE_SPECTRUM\n%--------------------------------------------------------------------------\nfile = path;\n%--------------------------------------------------------------------------\n\nif CHB\n    file_captrim = 'chip2_chb_cap.mat';\nelse\n    file_captrim = 'chip2_cha_cap.mat';\nend % CHB\n%--------------------------------------------------------------------------\n\n%Initial s port\ns         = serial('COM3');     % need to change if com number changes\ns.InputBufferSize = 128e3;\nset(s,'BaudRate',921600);\nfopen(s);\n\n\nif ANALYZE_SPECTRUM\n\n    if DATA_WRITE\n%        fifo_data = fifo_read(s, fifo_len);\ncommand = sprintf('fifo rst\\n');\nfwrite(s, command);\nfprintf('%s',command);\npause(0.1);\ncommand = sprintf('fifo rst\\n');\nfwrite(s, command);\nfprintf('%s',command);\npause(0.1);\ncommand = sprintf('fifo status\\n');\nfwrite(s,command);\nfprintf('%s',command);\npause(0.03);\ncommand = sprintf('fifo wr\\n');\nfwrite(s,command);\npause(1);\ncommand = sprintf('fifo status\\n');\nfwrite(s,command);\npause(0.03);\ncommand = sprintf('fifo read 0x%s\\n',dec2hex(fifo_len,2));\nfwrite(s,command);\npause(0.03);\n\npause(0.03);\nnum1 = s.BytesAvailable;\n\ndata_buffer = int8(zeros(1,fifo_len*1e3*30+500));\nfprintf(1,'Read fifo(%dK).',fifo_len);\n\nii = 1;\nwhile num1 ~= 0\n    pause(0.1);    \n    read_data = fread(s, num1);\n    data_buffer(ii:ii+num1-1) = read_data';\n    ii = ii + num1;\n    num1 = s.BytesAvailable;\n    fprintf(1,'.');\n%     fprintf(1,'%d\\n',ii);\nend\n\nfprintf(1,'\\n');\nfifo_data = data_buffer;\n\n       fprintf(1,'---------------------Read fifo ok!------------------------------\\n');\n       fid = fopen(file,'w');\n       fprintf(fid,'%1c',fifo_data);\n       fclose(fid);\n    end\n\n    fclose(s);\n%--------------------------------------------------------------------------\n    if DATA_LOAD\n    % read from data file\n    fid      = fopen(file,'r');\n    temp     = fscanf(fid, '%s'); \n    len_temp = length(temp);\n\n    for ii = 1:1:3000\n       if strcmp(temp(ii:ii+9),'fiforead0x')\n           break;\n       end\n    end\n\n    temp1              = temp(ii+12:fifo_len*16*1024+ii+11);\n    num_of_samples     = length(temp1)/16;\n\n    samples_rising_a   = zeros(1,num_of_samples);\n    samples_falling_a  = zeros(1,num_of_samples);\n\n    samples_rising_b   = zeros(1,num_of_samples);\n    samples_falling_b  = zeros(1,num_of_samples);\n\n    for ii = 1:1:num_of_samples\n        temp_rising_a  = temp1(((ii-1)*16+1):((ii-1)*16+4));\n        temp_falling_a = temp1((ii-1)*16+5:(ii-1)*16+8);\n        temp_rising_b  = temp1((ii-1)*16+9:(ii-1)*16+12);\n        temp_falling_b = temp1((ii-1)*16+13:(ii-1)*16+16);\n\n        samples_rising_a(ii)   = hex2dec(temp_rising_a);\n        samples_falling_a(ii)  = hex2dec(temp_falling_a);\n        samples_rising_b(ii)   = hex2dec(temp_rising_b);\n        samples_falling_b(ii)  = hex2dec(temp_falling_b);\n\n        if samples_rising_a(ii) > 2^13-1\n            samples_rising_a(ii) = samples_rising_a(ii) - 2^14;\n        end\n\n        if samples_rising_b(ii) > 2^13-1\n            samples_rising_b(ii) = samples_rising_b(ii) - 2^14;\n        end\n\n        if samples_falling_a(ii) > 2^13-1\n            samples_falling_a(ii) = samples_falling_a(ii) - 2^14;\n        end\n\n        if samples_falling_b(ii) > 2^13-1\n            samples_falling_b(ii) = samples_falling_b(ii) - 2^14;\n        end\n    end\n\n    mean_rising_a   = round(mean(samples_rising_a));\n    mean_falling_a  = round(mean(samples_falling_a));\n    mean_rising_b   = round(mean(samples_rising_b));\n    mean_falling_b  = round(mean(samples_falling_b));\n    end \n\n    fclose all;\n%--------------------------------------------------------------------------\n\n% % plot data\n% figure('name','sampled waveform');\n% \n% subplot(2,2,1); \n% plot(samples_rising_a); \n% title('ADC VI output'); \n% grid on;\n% hold on;\n% \n% subplot(2,2,2);\n% plot(samples_falling_a);\n% title('ADC VQ output');\n% grid on;\n% hold on;\n% \n% subplot(2,2,3); \n% plot(samples_rising_b);\n% title('ADC HI output');\n% grid on;\n% hold on;\n% \n% subplot(2,2,4);\n% plot(samples_falling_b);\n% title('ADC HQ output');\n% grid on;\n% hold on;\n%--------------------------------------------------------------------------\n\n% do fft analysis\nif FFT\n\n    if CHB    % CHB\n        dataI = samples_rising_b';\n        dataQ = samples_falling_b';\n        \n        if NCO\n            if DATA_IQ\n                data  = dataI - j*dataQ;\n            else\n                data  = dataQ - j*dataI;\n            end\n        else\n            data  = dataQ;\n        end\n        \n    else      % CHA\n        dataI = samples_rising_a';\n        dataQ = samples_falling_a';\n   \n        if NCO\n            if DATA_IQ\n                data  = dataI - j*dataQ;\n            else\n                data  = dataQ - j*dataI;\n            end\n        else\n            data  = dataQ;\n        end\n    end\n\n    if NF_TEST\n        len  = length(data); \n        fs   = 125e6; \n        fsig = 5e6;\n        t    = 1/fs:1/fs:len/fs; \n        %sig  = 8191*cos(2*pi*t*fsig);\n        sig  = 8191*cos(2*pi*t*fsig) + j * 8191*cos(2*pi*t*fsig);\n        data = data + sig';\n    end\n    \n    if SPUR340\n        len  = length(data); \n        fs   = 125e6; \n        fsig = 20e6;\n        t    = 1/fs:1/fs:len/fs;\n        amp  = 8191 * 10^(-59.2198/20);\n        td   = 0 ;\n        phase = 0.0717;\n        %sig  = 8191*cos(2*pi*t*fsig);\n        sig  = amp*cos(2*pi*(t+td)*fsig+phase) - j * amp*sin(2*pi*(t+td)*fsig+phase);\n        win  = hanning(len);\n        data_fft  =  fft(data.*win);\n        sig_fft   =  fft(sig'.*win);\n        abs(data_fft(5244))\n        abs(sig_fft(5244))\n        angle(data_fft(5244))\n        angle(sig_fft(5244))\n        %data = data - sig';   \n    end\n    \n    save fftdata.dat data -ASCII\n\n%     Dynamics_14b_no_print;\n%Filename:   Dynamics_12b.m\n%Function:   Spectrum analaysis of 12b ADC\n%Author:     Maxgress\n%Date:       Dec. 2012\n%--------------------------------------------------------------------------\n\n%set constants\n%--------------------------------------------------------------------------\n\n%fsample  = 61.44e6*4;           % clock frequency\nfsample  = 500e6/4;           % clock frequency\nfsr      = 1;\n%numpts   = 131072*2;          % 128k data\nnumpts   = 4096;            % 128k data\nnumbits  = 14;              % 12bit \nsearch   = 1;                      \nnumharm  = 3;              % Number of harmonics \n\n\n%load data\n%--------------------------------------------------------------------------\n\n%load C:\\MG6802\\fftdata.dat;\n%load fftdata.dat\n\n%data     = fftdata;\n[a b]    = size(data);\nnumpts   = a;\nwindow   = 1;\ntwotone  = 0;\ndither   = 0;\n\n%dBFS     = 20*log10((max(real(data))-min(real(data)))/2^numbits);\ndBFS     = 10*log10(((max(real(data))-min(real(data)))/2^numbits)^2 + ((max(imag(data))-min(imag(data)))/2^numbits)^2);\n\ntmp1     = size(data);\ntmp1     = tmp1(1);\n\n%process data\n%--------------------------------------------------------------------------\n\nq        =  data;\nfbin     = (fsample/numpts);\t%this is the the FFT bin spacing\nVopp     =  max(q)-min(q);\t%this is the Peak-to-Peak ADC output\nVodbfs   =  20*log10(Vopp/2);\t%this is the ADC output in dBFS\nshift    =  (2^(numbits-1))-0.5;\nu        =  (q-shift)/shift;\n\nz        =   fft(u)/numpts;\n\n%%%%%%%%% Here are some magic windowing factors \n\nif window==1;\n   a0=0.3635819;\n   a1=0.4891775;\n   a2=0.1365995;\n   a3=0.0106411;\n   vec=0.5*[-a3 a2 -a1 2*a0 -a1 a2 -a3]*(numpts/2^numbits);\n   winh=conv(vec,z);\n   for i=1:numpts;\n\t\tz(i)=winh(i+3);\n   end;\n\t\t\nend;\nGwin=-20*log10(a0);\t     %this is the window's gain\n\n%%%%%%%%%  these simple transforms are how we use the fft result:\n\nvolts=abs(z(1:(numpts/2+1)));\n%volts(numpts/4:numpts/2+1)=0.00001;\n\npower=volts.^2;\ndbvolts=20*log10(2*volts+eps); % Why the factor of 2 applied to volts.\n%dbvolts(numpts/4:numpts/2+1)=-92;\nif window==1;\n\tdbvolts=dbvolts+Gwin;\t%this resets to normalized gain\nend;\ndbint=floor(dbvolts);\n\n%  if the oscillator frequencies are all over the place,\n%  we can go and find the input by looking for the max \n%  bin.  This is selected by the \"search\" flag.\n\nif search==1\n\ttempvolts=volts;\n\ttempvolts(1:4)=zeros(1,4);\n\t[a1,fund]=max(tempvolts);\n   finput=(fund-1)*fsample/numpts;\n   tempvolts(fund)=0;\n   if(twotone==1)\n      [a2,fundq]=max(tempvolts);\n      finputq=(fundq-1)*fsample/numpts;\n   end;   \nend;\n\n%%%%%%%%%%%%%  Now we analyze the results of the fft;\n%%%%%%%%%%%%%  If we know finput, we can find the harmonics:\nif(twotone==1)\nhq=0:(numharm-1);\nfhq=finputq*hq;\nrbinsq=round(fhq/(fsample/numpts));\nmultq=(floor(rbinsq/(numpts/2)));\npolq=(-1).^multq;\nactbinq=1+(numpts/2)*(1-polq)/2+polq.*(rbinsq-multq*numpts/2);\nfor i=1:numharm;\n      hdarrayq(i)=dbvolts(actbinq(i));\nend;\nend;\n\nh=0:(numharm-1);\nfh=finput*h;\nrbins=round(fh/(fsample/numpts));\nmult=(floor(rbins/(numpts/2)));\npol=(-1).^mult;\nactbin=1+(numpts/2)*(1-pol)/2+pol.*(rbins-mult*numpts/2);\ndbvoltsa=dbvolts;\n\nfor i=1:numharm;\n  \n      hdarray(i)=dbvolts(actbin(i));\n\nend;\n\n%%%%%%% After calculating harmonic bin locations, we can calculate the\n%%%%%%% noise floor for the SNR & SINAD. First exclude the power in the  \n%%%%%%% dither (this is the \"dither\" variable) band and the 50 individual\n%%%%%%% harmonic bins and the DC bin. An iterative approach is used.\n%%% actbin(1) is DC bin.  \n%%% actbin(2) is the fundamental.\n\nif dither>0\n\tpbins=power;\n\tstartBin=dither/fbin;\n\tavgpwr1=sum(pbins(startBin+1):pbins(startBin+5));\n\tfor i=1:startBin;\n\t\tpbins(i)=avgpwr1;\n\tend;\nelse\n\tpbins=power;\nend;\nsfdrarray=pbins;\nzeroset=0;\npowleng=1+length(power);\nvart=8;\nif window==0\n   \tfor i=1:numharm;\n         pbins(actbin(i))=0;\n         if(twotone==1)\n            pbins(actbinq(i))=0;\n         end;\n      end;\n\t\t\tavgpwr2=mean(pbins)*((numpts/2)+1)/((numpts/2)-(numharm)+1);\n\t\n   %%%%% Commenting out code which fills harmonic bins with average\n   %%%%% power with window == 0.\n%\tfor i=1:numharm;\n%\t\tpbins(actbin(i))=avgpwr2;\n%\tend;\n\n%%% this next bunch of loops deal with the window's sidelobes\nelse\n\tfor i=1:numharm;\n\t\tif (actbin(i)-4) >  0;\n\t\t\tpbins(actbin(i)-4)=0;\n\t\t\tzeroset=zeroset+1;\n\t\t\tend;\n\t\tif (actbin(i)-3) >  0;\n\t\t\tpbins(actbin(i)-3)=0;\n\t\t\tzeroset=zeroset+1;\n\t\t\tend;\n\t\tif (actbin(i)-2) >  0;\t\n\t\t\tpbins(actbin(i)-2)=0;\n\t\t\tzeroset=zeroset+1;\n\t\t\tend;\n\t\tif (actbin(i)-1) >  0;\t\n\t\t\tpbins(actbin(i)-1)=0;\n\t\t\tzeroset=zeroset+1;\n\t\t\tend;\n\t\tpbins(actbin(i))=0;\n\t\tzeroset=zeroset+1;\n\t\tif (actbin(i)+1) < powleng\n\t\t\tpbins(actbin(i)+1)=0;\n\t\t\tzeroset=zeroset+1;\n\t\t\tend;\n\t\tif (actbin(i)+2) < powleng\n\t\t\tpbins(actbin(i)+2)=0;\n\t\t\tzeroset=zeroset+1;\n\t\t\tend;\n\t\tif (actbin(i)+3) < powleng\n\t\t\tpbins(actbin(i)+3)=0;\n\t\t\tzeroset=zeroset+1;\n\t\t\tend;\n\t\tif (actbin(i)+4) < powleng\n\t\t\tpbins(actbin(i)+4)=0;\n\t\t\tzeroset=zeroset+1;\n\t\t\tend;\n\tend;\n\tavgpwr2=mean(pbins)*(numpts+1)/((numpts)-3-zeroset);\nend;\n\nif dither>0\n\tfor i=1:startBin;\n\t\tpbins(i)=avgpwr2;\n\tend;\nend;\n\nif(window==1)\n\tfor i=1:numharm;\n\t\tif (actbin(i)-4) >  0;\n\t\t\tpbins(actbin(i)-4)=avgpwr2;\n\t\tend;\n\t\tif (actbin(i)-3) >  0;\n\t\t\tpbins(actbin(i)-3)=avgpwr2;\n\t\tend;\n\t\tif (actbin(i)-2) >  0;\t\n\t\t\tpbins(actbin(i)-2)=avgpwr2;\n\t\tend;\n\t\tif (actbin(i)-1) >  0;\t\n\t\t\tpbins(actbin(i)-1)=avgpwr2;\n\t\tend;\n\t\tpbins(actbin(i))=avgpwr2;\n\t\tif (actbin(i)+1) < powleng\n\t\t\tpbins(actbin(i)+1)=avgpwr2;\n\t\tend;\n\t\tif (actbin(i)+2) < powleng\n\t\t\tpbins(actbin(i)+2)=avgpwr2;\n\t\tend;\n\t\tif (actbin(i)+3) < powleng\n\t\t\tpbins(actbin(i)+3)=avgpwr2;\n\t\tend;\n\t\tif (actbin(i)+4) < powleng\n\t\t\tpbins(actbin(i)+4)=avgpwr2;\n\t\tend;\n\tend;\n    %if (actbin(2)-4 < 1) low_lim = 1; else low_lim = actbin(2) - 4; end\n    %if (actbin(2)+4 > length(power)) high_lim = length(power); else high_lim = actbin(2) + 4; end\n    \n    if (actbin(2)- 128 < 1) low_lim = 1; else low_lim = actbin(2) - 128; end\n    if (actbin(2)+ 128 > length(power)) high_lim = length(power); else high_lim = actbin(2) + 128; end\n    \n\tfundpower=sum(power(low_lim:high_lim));\n\tsnr=10*log10(fundpower/sum(pbins));\n\thdarray';\nend;\n\n\n% This one calculates the ADC's thermal noise floor w.r.t. FSR\n%\t\"Gwin\" is the reciprocal of the window's gain\nif window==1\n\tGwin=-1*(20*log10(a0));\nelse\n\tGwin=0;\nend;\nGfft=10*log10(numpts);\nnoisefloor=Gfft + 20*log10(avgpwr2^.5) + Gwin;\n\nif(window==0)\n   if(twotone==1)\n      fundpower=power(actbin(2))+power(actbinq(2));\n   else\n      fundpower=power(actbin(2));\n   end;\n   if(ericsson==1)\n      snr=10*log10(fundpower/sum(pbins(1:1024)))\n   else\n      snr=10*log10(fundpower/sum(pbins))\n   end;\n   \n\thdarray';\nend;\n\nfundampl=hdarray(2);\n\n\n%  Now we use the sfdrarray generated above, remove the fundamental and\n%  bins, and look for\n%  the next largest bin.  We calculate SFDR, then output a number showing\n%  the dominant harmonic\n%  0 will represent a non-harmonic spur...\n\nsfdrarray(1)=0;\nsfdrarray(actbin(2))=0;\nif(twotone==1)\n   sfdrarray(actbinq(2))=0;\nend;\nif window==1;\n\tsfdrarray(1:4)=zeros(1,4);\n\tsfdrarray(low_lim:high_lim)=zeros(1,high_lim-low_lim+1);\nend;\nsfdr_ray=sfdrarray;\n \n[a,sfdrbin]=max(sfdr_ray);\nsfdrbin;\nsfdr=10*log10((power(actbin(2)))/a);\ndomharm=0;\nfor i=3:numharm;\n\tif actbin(i)==sfdrbin;\n\t\tdomharm=i-1;\n\tend;\nend;\ndomharm;\nspurfreq=(sfdrbin-1)*fsample/numpts;\n\n%%%%   SINAD calculation\n%%%%  I think that it is valid to eliminate the dc bin for calculating SINAD.\n%%%%  I need to check\n%%%%  to see if everyone else agrees with this.\n\nif window==0\n\t% sfdrarray(1)=avgpwr2; %Add average noise power to DC bin.\n   if(ericsson==1)\n      allnoise=sum(sfdrarray(1:1024));\n   else\n      allnoise=sum(sfdrarray);\n   end;\n   if(twotone==1)\n      sinad=10*log10((power(actbin(2))+power(actbinq(2)))/allnoise);\n   else\n      sinad=10*log10(power(actbin(2))/allnoise);\n   end;\n   \nelse\n\tsfdrarray(1:4)=avgpwr2*ones(1,4);\n\tallnoise=sum(sfdrarray);\n\tsinad=10*log10(fundpower/allnoise);\nend;\n\nwinharm=[];\n\nif(window==1)\n   winfund=power(low_lim:high_lim);\n   for i=3:numharm;\n      winharm=[winharm power(low_lim:high_lim)'];\n   end;\n   thd=10*log10(sum(winfund)/sum(sum(winharm)));\nelse\n   \n%   Now we want to calculate THD (in dBc).  This is just:\n%Need total Harmonic calculation for window == 1.\n\n\ttotharm=0;\n\tfor i=3:numharm;\n      if(ericsson==1)\n      \tif(actbin(i)>1024)\n         \ttotharm=totharm;\n      \telse\n         \ttotharm=totharm+power(actbin(i));\n      \tend;\n   \telse\n      \ttotharm=totharm+power(actbin(i));\n   \tend;\n\tend;\n\tthd=10*log10(power(actbin(2))/totharm)\n\nend;\n\n%%%%%%%%%%  To check the calculations, I compared the sum of thd and snr to the\n%%%%%%%%%%  sinad=\n%%%%%%%%%%   calculated.  They work out quite closely with various input SNR's.\n\nsinad2=10*log10(1/(10^(thd/10))+1/(10^(snr/10)));\nsinad+sinad2;\n\n%%%%%%%%  ENOB calculation: \n\nenob=(sinad-1.760912)/6.0206;\nHD2=dbvolts(actbin(2))-dbvolts(actbin(3));\n% HD3=dbvolts(actbin(2))-dbvolts(actbin(4));\n\n%  One final calculation: dc offset in mv\n%  note that fsr is the full scale range (peak to peak) in volt\noffset=mean(data);\nxax=fbin*(1:1:numpts/2+1);\nspectrum=dbvolts(10:length(dbvolts));\nspectrum=dbvolts-max(spectrum);\n%offset, fundampl, snr, sfdr, thd, sinad, noisefloor\n\n\n\n    if CHB\n        fprintf(1,'CHB analys \\n dBFs=%4.2fdB  SNR=%4.2fdB  SFDR=%4.2fdB  SINAD=%4.2fdB \\n THD =  %4.2fdB  ENOB=%4.2fbits  OFFSET=%4.2fLSBS\\n',dBFS,snr,sfdr,sinad,thd,enob,offset);\n    else\n        fprintf(1,'CHA analys \\n dBFs=%4.2fdB  SNR=%4.2fdB  SFDR=%4.2fdB  SINAD=%4.2fdB \\n THD =  %4.2fdB  ENOB=%4.2fbits  OFFSET=%4.2fLSBS\\n',dBFS,snr,sfdr,sinad,thd,enob,offset);\n    end\n\nfigure('name','frequency_spectrum');\n\n    freq = linspace(0,numpts/2,numpts/2+1)/numpts * fsample/1e6;\n\nplot(freq,spectrum);\n\nfre_spectrum=spectrum';\n\n    if CHB\n        title('ADC CHB output spectrum(H)'); \n    else\n        title('ADC CHA output spectrum(V)');\n    end\n\nxlabel('Freq(MHz)'); \nnote = sprintf('SNR = %5.2fdB\\nSFDR = %5.2fdB\\ndBFS = %5.2fdB\\n',snr,sfdr,dBFS);\ntext(max(freq)/2,max(spectrum)-30,note);\ngrid on;\n\ntime=datestr(now,'yyyymmddTHHMMSS');\nsaveas(gcf,[path_jpg,'A_',frequency,vol13,vol20,'_',time],'jpg');\n\nfprintf(1,'---------------------FFT analysis done!-------------------------\\n');\n\nend  % if FFT\nelse\nfclose(s);\nend  % if ANALYZE_SPECTRUM\n%--------------------------------------------------------------------------\n\nif ANALYZE_INL\n    DNLINL_14b;\n    figure;\n    plot(INL);\n    fprintf(1,'---------------------INL analysis done!-------------------------\\n');\nend\n%--------------------------------------------------------------------------\n%--------------------------------------------------------------------------"("??"=w114, "ANALYZE_SPECTRUM"=1.0 ("Real"), "DATA_WRITE"=1.0 ("Real"), "DATA_LOAD"=1.0 ("Real"), "CHB"=1.0 ("Real"), "FFT"=1.0 ("Real"), "NCO"=0.0 ("Real"), "DATA_IQ"=w90, "NF_TEST"=0.0 ("Real"), "SPUR340"=1.0 ("Real"), "ANALYZE_INL"=0.0 ("Real"), "path"=w111, "path_jpg"=w112, "frequency"=w126, "vol13"=w127, "vol20"=w128) -> ("??"=w110:errorcluster, "freq"=w116:dbl[], "fre_spectrum"=w115:dbl[], "dBFS"=w86:dbl, "snr"=w85:dbl, "sfdr"=w84:dbl)  [unwired: 4 out]
          n93 = Bundle(w116, w115) -> (→"XY Graph 2":cluster{dbl[], dbl[]})  [unwired: 1 in]
          n94 = Build Array(w86, w85, w84) -> (w83:dbl[])
          "parameters_b" <- w83
        }
        n95 = Open VI Reference(type specifier VI Refnum (for type only)=refnum<vi> refnum, vi path=path "C:/Users/pigandhome/Desktop/Everst_LV2015/save_rx.vi") -> (vi reference=w65:refnum<vi>, error out=w64:errorcluster)  [unwired: 4 in]
        n96 = Array Size(array=w60) -> (size(s)=w59:i32)
        n97 = Path To String(path=w55) -> (string=w54:string)
        n98 = call-by-ref "?"(reference=w65, error in=w64, "PA"=w58, "PB"=w57, "PATH"=w54, "Tabsize"=w59, "FreqTab"=w60) -> (reference out=w61:refnum<vi>, error out=w62:errorcluster)  [unwired: 15 in]
        n99 = Close Reference(reference=w61, error in (no error)=w62) -> ()  [unwired: 1 out]
      }
    }
  }
